vi "FTW-XML-Destroy.vi"(0 "XML Node":refnum<k20>, 11 "error in":errorcluster) -> (15 "error out":errorcluster)   [LabVIEW 2013, in "XML.lvlib"]
uses:
  XML.lvlib
  DOMDefRefCommand.ctl
panel:
  # "Inputs"
  # "Outputs"
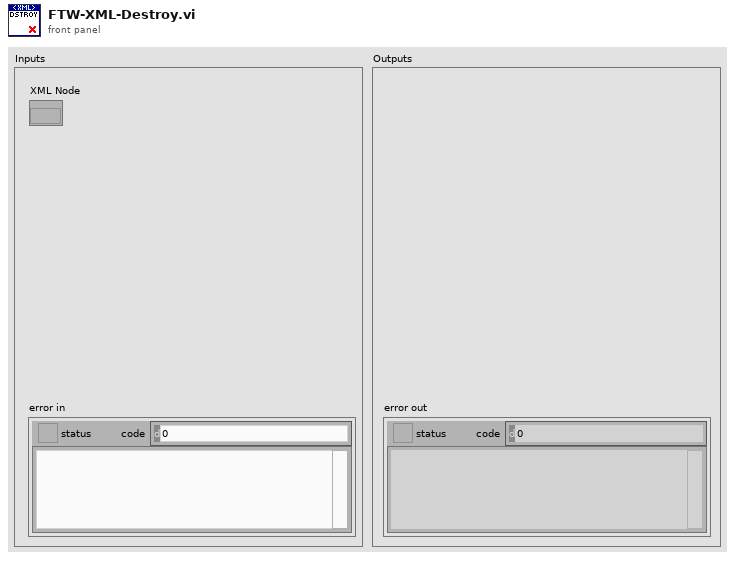
[diagram p1: front panel]
types:
  T1 = typedef "DOMDefRefCommand.ctl" = enum16{"No Command - Error", "Initialise", "Open Document", "Allocate RefNum", "Close Document"}
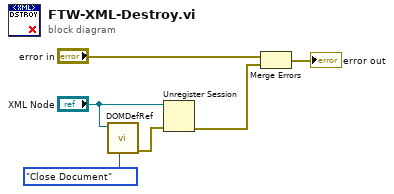
[diagram p0: block diagram]
diagram:
  n1 = call "DOMDefRef.vi"("DOMUserDefRefCommand"=DOMDefRefCommand."Close Document", "Refnum in"="XML Node") -> ("error out"=w2:errorcluster)  [unwired: 4 in, 2 out]
  n2 = Unregister Session(8:w2, 11:"XML Node") -> (0:w4:errorcluster)
  n3 = Merge Errors("error in", w4) -> (→"error out":errorcluster)
